vi "Recalculate Toolbar Width.vi"(8 "error in (no error)":errorcluster, 11 "Toolbar Control in":refnum<class "Toolbar Control.lvclass">) -> (0 "error out":errorcluster, 3 "Toolbar Control out":refnum<class "Toolbar Control.lvclass">)   [LabVIEW 2011, in "Toolbar Control.lvclass"]
doc: "This VI will calculate the Toolbar Width, of a vertical toolbar based on the icon size, and the icon names provided. This information is then stored in the object data.\n\n-------------\nDeveloped by Brian Hoover (hooovahh)"
uses:
  Toolbar Control.lvclass
  Toolbar Control.lvclass/Toolbar Control.ctl
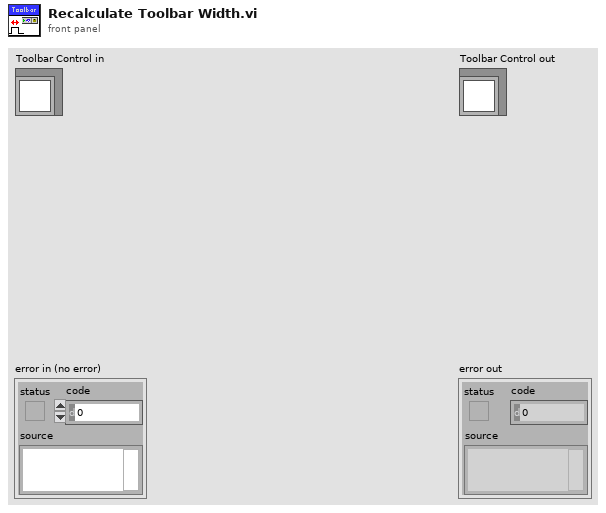
[diagram p1: front panel]
types:
  T1 = enum16{"User-specified Font", "Application Font", "System Font", "Dialog Font"}
  T2 = typedef "Toolbar Control.lvclass/Icon Data.ctl" = cluster{"Original Image Path":path, "Original Image Data":T3, "Scaled Icon":picture, "Button Name":string, "Button State":T4, "Icon Type":T5}
  T3 = typedef "imagedata.ctl" = cluster{"image type":i32, "image depth":i32, "image":u8[], "mask":u8[], "colors":u32[], "Rectangle":cluster{"left":i16, "top":i16, "right":i16, "bottom":i16}}
  T4 = typedef "Toolbar Control.lvclass/Button State.ctl" = enum8{"Enabled", "Disabled", "Disabled and Grayed Out"}
  T5 = typedef "Icon Type.ctl" = enum16{"Normal Icon", "Separator Icon", "More Options"}
  T6 = cluster{"left":i16, "top":i16, "right":i16, "bottom":i16}
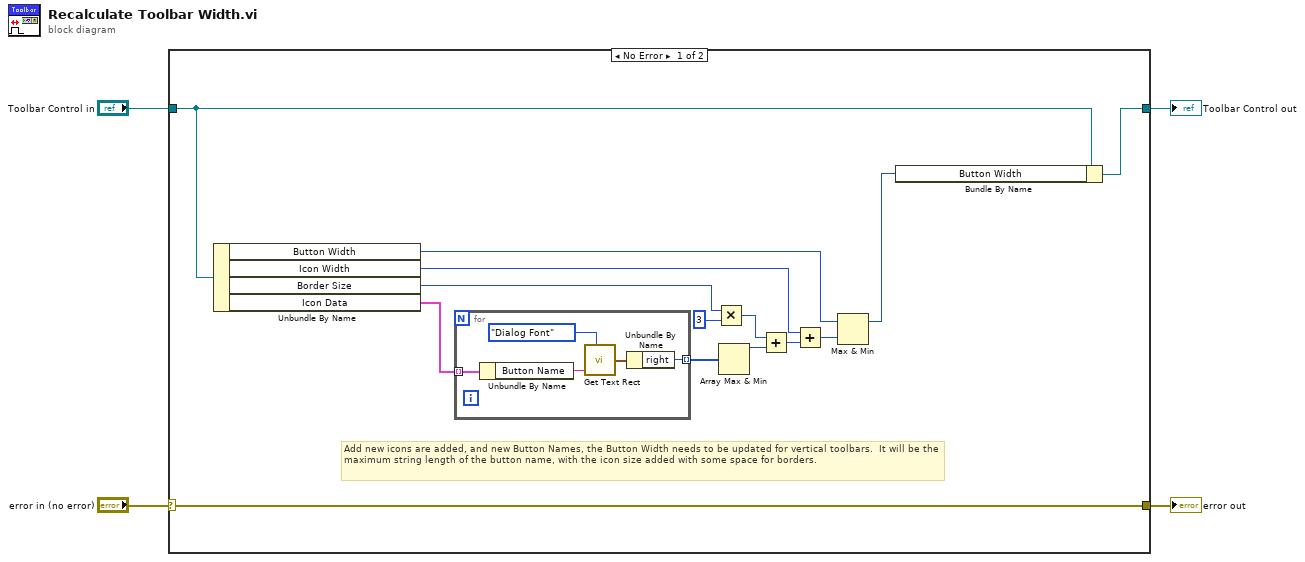
[diagram p0: block diagram]
diagram:
  n1 = case shown="No Error" "error in (no error)" {
    selector: "error in (no error)" -> [w18 w25]
    tunnel: [w18 w25] -> w3
    tunnel: [w17 w24] -> w1
    tunnel: "Toolbar Control in" -> [w9 w24]
    frame No Error {
      # "Add new icons are added, and new Button Names, the Button Width needs to be updated for vertical toolbars.  It will be the maximum string length of the button name, with the icon size added with some space for borders."
      n2 = Unbundle By Name(w9) -> ("Button Width"=w6:i32, "Icon Width"=w16:i32, "Border Size"=w8:i16, "Icon Data"=w15:T2[])
      n3 = for {
        tunnel: w15 -> [w23] mode=indexing
        tunnel: [w20] -> w10 mode=indexing
        n4 = Unbundle By Name(w23) -> ("Button Name"=w22:string)
        n5 = call <vilib>:"Get Text Rect.vi"("desired font(Application)"=T1."Dialog Font", "text"=w22) -> ("rect"=w21:T6)  [unwired: 7 in]
        n6 = Unbundle By Name(w21) -> ("right"=w20:i16)
      }
      n7 = Multiply(x=w8, y=i16 3) -> (x*y=w13:i16)
      n8 = Array Max & Min(array=w10) -> (max value=w14:i16)  [unwired: 3 out]
      n9 = Add(x=w13, y=w14) -> (x+y=w11:i16)
      n10 = Add(x=w16, y=w11) -> (x+y=w7:i32)
      n11 = Max & Min(x=w6, y=w7) -> (max(x,y)=w5:i32)  [unwired: 1 out]
      n12 = Bundle By Name(cluster=w9, "Button Width"=w5) -> (w17:refnum<class "Toolbar Control.lvclass">)
    }
    frame Error {
    }
  }
  "error out" <- w3
  "Toolbar Control out" <- w1
